vi "Reslut.vi"() -> ()   [LabVIEW 2018]
panel:
  out "ResultOut":T1
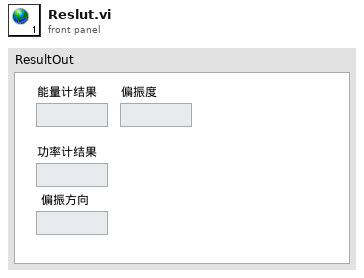
[diagram p1: front panel]
types:
  T1 = cluster{"能量计结果":string, "功率计结果":string, " 偏振方向":string, "偏振度":string}
diagram:
